vi "_Show Wire Label.vi"(6 "Variant in":variant=variant(cluster{"FP.IsFrontMost?":bool, "Project VI Path":path, "Palette Object Name":string} {"FP.IsFrontMost?"=FALSE, "Project VI Path"=path "", "Palette Object Name"=""}), 8 "error in (no error)":errorcluster, 9 "Shift Pressed?":bool, 10 "QD Combo Box Ref":refnum<vi>, 11 "QD Launch VI Ref":refnum<vi>) -> (0 "error out":errorcluster, 4 "Variant out":variant=variant(bool TRUE))   [LabVIEW 2014, in "NEVSTOP QD Shortcuts.lvlib"]
uses:
  NEVSTOP QD Shortcuts.lvlib
panel:
  in  "Undo Name":string="NEVSTOP_Show Wire Label"
  # "Do not change the connector pane of this VI.\n\nSee the block diagram for directions on how to use this template."
  # "Specify the name of the Undo transaction"
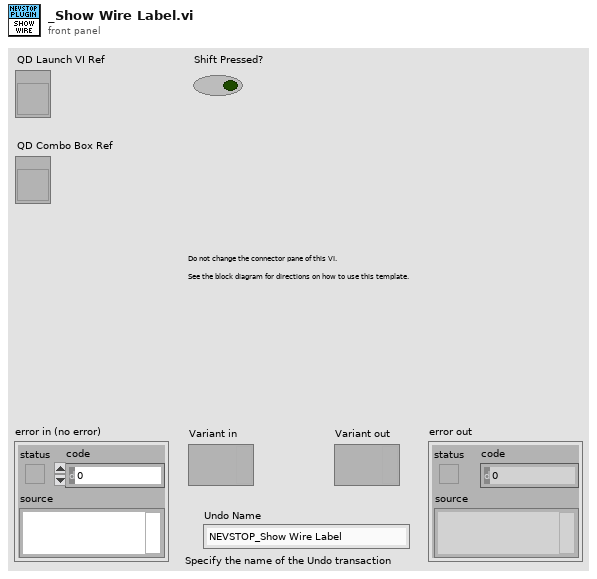
[diagram p1: front panel]
types:
  T1 = typedef "LVPositionTypeDef.ctl" = cluster{"Left":i32, "Top":i32}
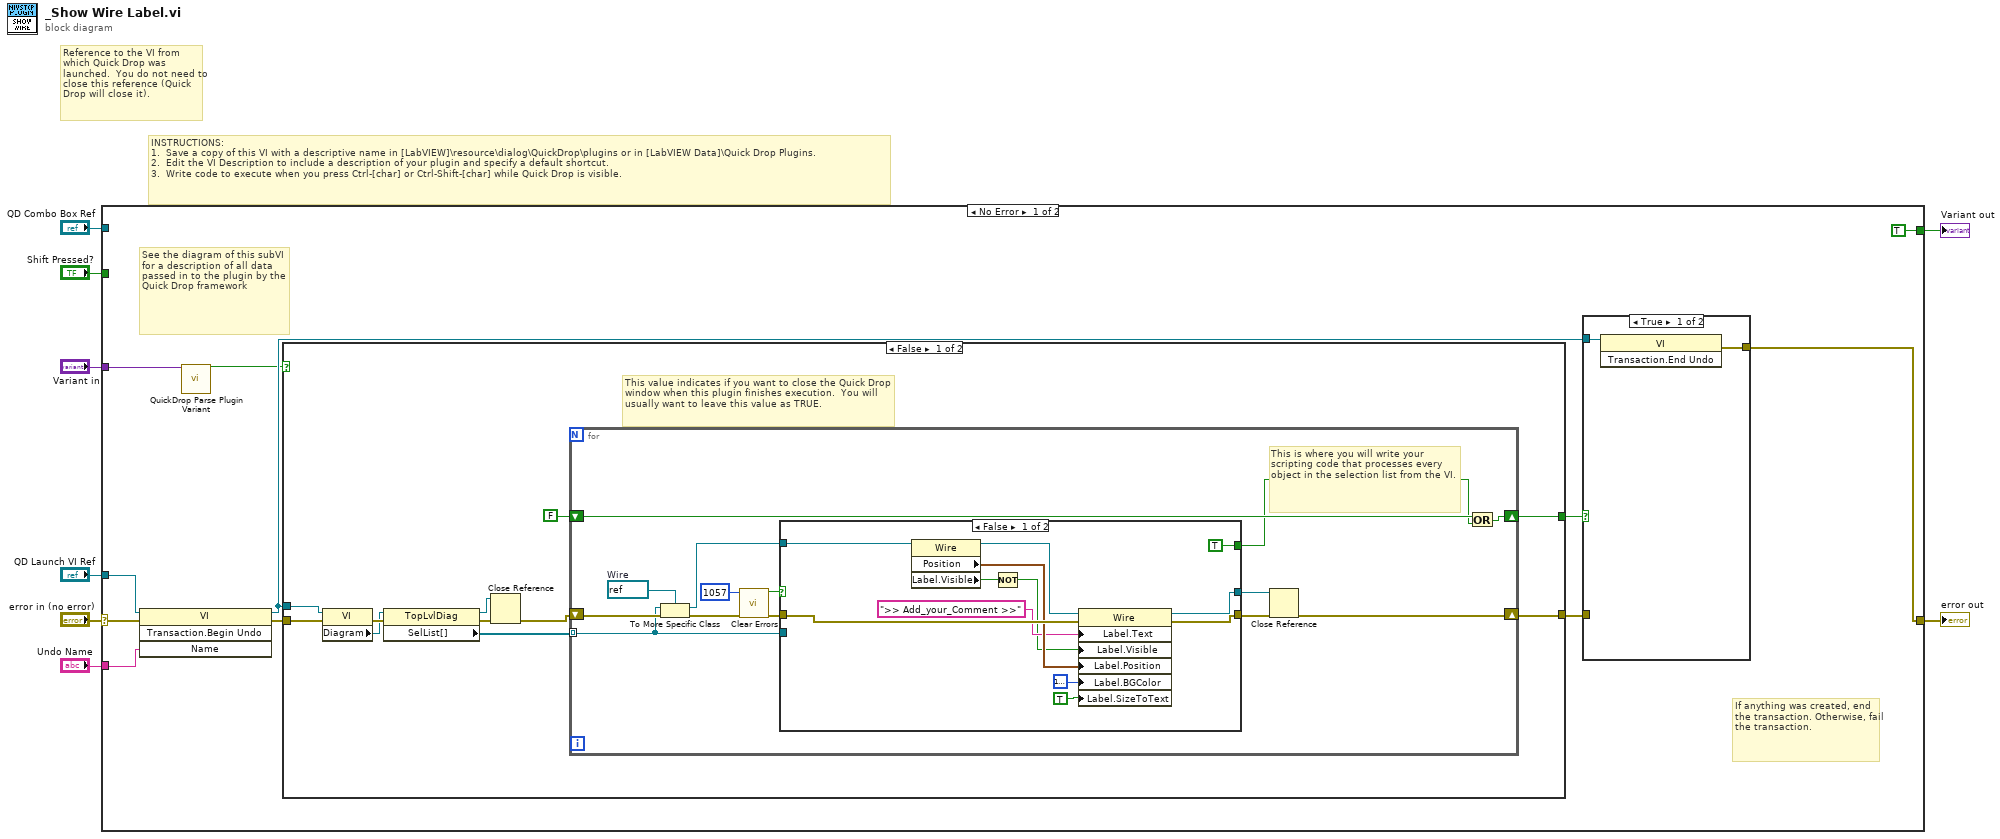
[diagram p0: block diagram]
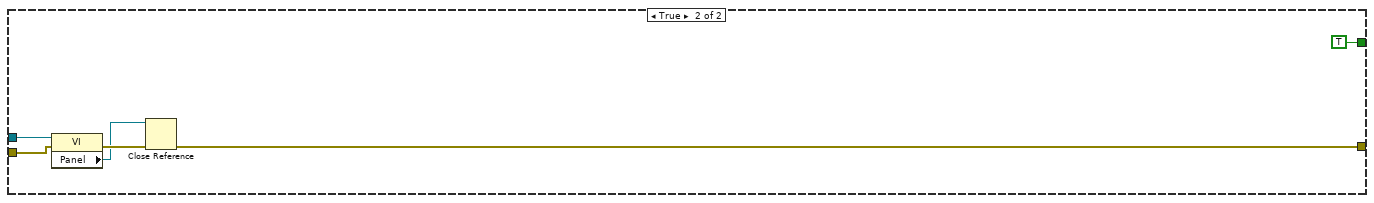
[diagram p3: hidden frame]
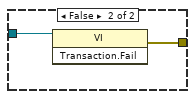
[diagram p4: hidden frame]
diagram:
  # "Reference to the VI from which Quick Drop was launched.  You do not need to close this reference (Quick Drop will close it)."
  # "INSTRUCTIONS:\n1.  Save a copy of this VI with a descriptive name in [LabVIEW]\\resource\\dialog\\QuickDrop\\plugins or in [LabVIEW Data]\\Quick Drop Plugins.\n2.  Edit the VI Description to include a description of your plugin and specify a default shortcut. \n3.  Write code to execute when you press Ctrl-[char] or Ctrl-Shift-[char] while Quick Drop is visible."
  n1 = case shown="No Error" "error in (no error)" {
    selector: "error in (no error)" -> [w18 w69]
    tunnel: [w13 w69] -> w7
    tunnel: "QD Launch VI Ref" -> [w17 _]
    tunnel: "Shift Pressed?" -> [_ _]
    tunnel: "QD Combo Box Ref" -> [_ _]
    tunnel: "Variant in" -> [w19 _]
    tunnel: "Undo Name" -> [w16 _]
    tunnel: [TRUE _] -> w1
    frame No Error {
      # "If anything was created, end the transaction. Otherwise, fail the transaction."
      # "See the diagram of this subVI for a description of all data passed in to the plugin by the Quick Drop framework"
      n2 = invoke class="VI" method="Transaction.Begin Undo"(reference=w17, error in=w18, "Name"=w16) -> (reference out=w11:refnum<vi>, error out=w14:errorcluster)  [unwired: 1 in, 2 out]
      n3 = call <vilib>:"QuickDrop Parse Plugin Variant.vi"("QDKS Variant in"=w19) -> ("QD Launch VI Panel?"=w9:bool)  [unwired: 12 in, 2 out]
      n4 = case shown="False" w9 {
        tunnel: w14 -> [w30 w61]
        tunnel: [w28 w60] -> w12
        tunnel: w11 -> [w27 w62]
        tunnel: [w25 TRUE] -> w10
        frame False {
          # "This value indicates if you want to close the Quick Drop window when this plugin finishes execution.  You will usually want to leave this value as TRUE."
          n5 = property class="VI"(reference=w27, error in=w30) -> (error out=w23:errorcluster, "Diagram"=w22:refnum<vi>)  [unwired: 1 out]
          n6 = property class="TopLvlDiag"(reference=w22, error in=w23) -> (reference out=w20:refnum<vi>, error out=w21:errorcluster, "SelList[]"=w24:refnum<vi>[])
          n7 = Close Reference(reference=w20, error in (no error)=w21) -> (error out=w29:errorcluster)
          n8 = for {
            shift-right: [w42] -> w28
            shift-left: w29 -> [w39]
            shift-right: [w43] -> w25
            shift-left: FALSE -> [w44]
            tunnel: w24 -> [w35] mode=indexing
            w41 = refnum<vi> refnum  # Wire
            # "This is where you will write your scripting code that processes every object in the selection list from the VI."
            n9 = To More Specific Class(target class=w41, reference=w35, error in=w39) -> (specific class reference=w36:refnum<vi>, error out=w40:errorcluster)
            n10 = call <vilib>:"Clear Errors.vi"("error in (no error)"=w40, "specific error code to clear (0: all)"=1057) -> ("error out"=w37:errorcluster, "specific error cleared?"=w33:bool)  [unwired: 4 in]
            n11 = case shown="False" w33 {
              tunnel: [w54 w58] -> w38
              tunnel: w37 -> [w53 w58]
              tunnel: w36 -> [w56 _]
              tunnel: w35 -> [_ w57]
              tunnel: [w55 w57] -> w34
              tunnel: [TRUE ("x") _] -> w32
              frame False {
                n12 = property class="Wire"(reference=w56) -> (reference out=w51:refnum<vi>, "Position"=w50:T1, "Label.Visible"=w47:bool)  [unwired: 1 in, 1 out]
                n13 = Not(x=w47) -> (.not. x?=w46:bool)
                n14 = property class="Wire"(reference=w51, error in=w53, "Label.Text"=">> Add_your_Comment >>", "Label.Visible"=w46, "Label.Position"=w50, "Label.BGColor"=u32 16777216 ("Label.Text Colors:BG Color"), "Label.SizeToText"=TRUE ("Label.Size to Text?")) -> (reference out=w55:refnum<vi>, error out=w54:errorcluster)
              }
              frame True {
              }
            }
            n15 = Close Reference(reference=w34, error in (no error)=w38) -> (error out=w42:errorcluster)
            n16 = Or(x=w44, y=w32) -> (x .or. y?=w43:bool)
          }
        }
        frame True {
          n17 = property class="VI"(reference=w62, error in=w61) -> (error out=w64:errorcluster, "Panel"=w63:refnum<vi>)  [unwired: 1 out]
          n18 = Close Reference(reference=w63, error in (no error)=w64) -> (error out=w60:errorcluster)
        }
      }
      n19 = case shown="True" w10 {
        tunnel: w11 -> [w65 w67]
        tunnel: [w66 w68] -> w13
        tunnel: w12 -> [_ _]
        frame True {
          n20 = invoke class="VI" method="Transaction.End Undo"(reference=w65) -> (error out=w66:errorcluster)  [unwired: 2 in, 2 out]
        }
        frame False {
          n21 = invoke class="VI" method="Transaction.Fail"(reference=w67) -> (error out=w68:errorcluster)  [unwired: 2 in, 2 out]
        }
      }
    }
    frame Error {
    }
  }
  "error out" <- w7
  "Variant out" <- w1
